vi "PosBolaFora.vi"(5 "AI Parameters":T1={"GotoKick"={"Dist do cone a frente"=150.0, "attacker farback"=1500.0, "Perto"=300.0, "min dist to kick"=150.0, "kick eps"=0.0, "Time to transition"=0.05}, "Attacker"={"CC chute"=0.09, "CC passe"=0.045, "Kick Force"=100.0, "ball-robot Kick"=200.0, "ball-robot Pass"=0.3, "drible\nAttk"=FALSE}, "Defender"={"D max"=1700.0, "Vel p/ robô av"=1000.0, "Kick Force"=100.0, "D atk-def"=0.0, "D farback"=0.0, "drible\ndef"=FALSE, "drible\ngoalie"=FALSE}, "Timeout"={"Field/v in x"=6.0, "Dist Robots"=300, "Dist up in y"=300}, "Pose Striker"={"dist"=200.0, "Numeric"=-4.0, "dist 2"=200.0, "drible\nstriker"=FALSE}, "Dist Stop"=300.0, "D ball out"=200, "D central gap "=150.0, "T pass"=0.0, "Force ++"=0.0, "range kick"=0.0, "Chute alto"=TRUE, "Marcador novo"=TRUE, "drible"=FALSE, "D drible"=300.0} {"D drible" format="%#_13g"; "D central gap" format="%#_13g"; "Dist Stop" format="%#_13g"; "Pose Striker"."Numeric" format="%#_13g"; "Defender"."Kick Force" format="%#_13g"; "Defender"."Vel p/ robô av" format="%#_13g"; "Attacker"."ball-robot Kick" format="%#_13g"; "Attacker"."Kick Force" format="%#_13g"; "Attacker"."CC passe" format="%#_13g"; "Attacker"."CC chute" format="%#_13g"; "GotoKick"."min dist to kick" format="%#_13g"; "GotoKick"."Perto" format="%#_13g"; "GotoKick"."attacker farback" format="%#_13g"; "GotoKick"."Dist do cone a frente" format="%#_13g"}, 9 "Field Size in":T2, 10 "Position da bola":dbl[](array[numeric]), 11 "Position do robot":dbl[](array[numeric])) -> (3 "Target":dbl[](array[numeric]))   [LabVIEW 2017]
uses:
  Core/Field Size.ctl
  AI Parameters.ctl
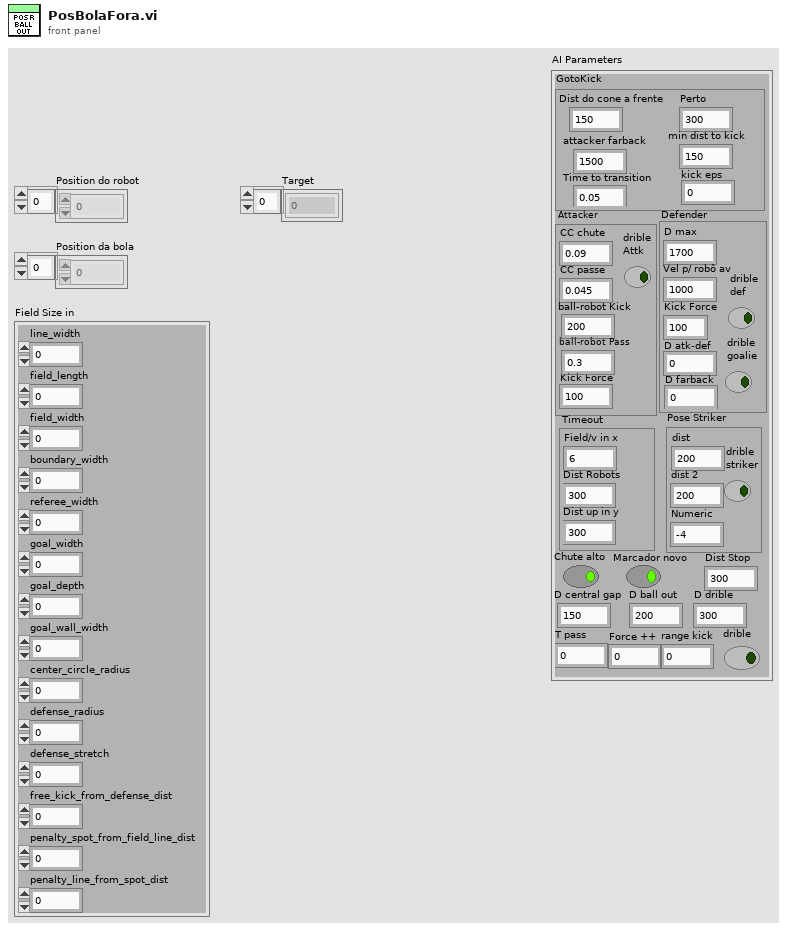
[diagram p1: front panel]
types:
  T1 = typedef "AI Parameters.ctl" = cluster{"GotoKick":cluster{"Dist do cone a frente":dbl, "attacker farback":dbl, "Perto":dbl, "min dist to kick":dbl, "kick eps":dbl, "Time to transition":dbl}, "Attacker":cluster{"CC chute":dbl, "CC passe":dbl, "Kick Force":dbl, "ball-robot Kick":dbl, "ball-robot Pass":dbl, "drible\nAttk":bool}, "Defender":cluster{"D max":dbl, "Vel p/ robô av":dbl, "Kick Force":dbl, "D atk-def":dbl, "D farback":dbl, "drible\ndef":bool, "drible\ngoalie":bool}, "Timeout":cluster{"Field/v in x":dbl, "Dist Robots":u32, "Dist up in y":u32}, "Pose Striker":cluster{"dist":dbl, "Numeric":dbl, "dist 2":dbl, "drible\nstriker":bool}, "Dist Stop":dbl, "D ball out":i32, "D central gap ":dbl, "T pass":dbl, "Force ++":dbl, "range kick":dbl, "Chute alto":bool, "Marcador novo":bool, "drible":bool, "D drible":dbl}
  T2 = typedef "Field Size.ctl" = cluster{"line_width":u32, "field_length":u32, "field_width":u32, "boundary_width":u32, "referee_width":u32, "goal_width":u32, "goal_depth":u32, "goal_wall_width":u32, "center_circle_radius":u32, "defense_radius":u32, "defense_stretch":u32, "free_kick_from_defense_dist":u32, "penalty_spot_from_field_line_dist":u32, "penalty_line_from_spot_dist":u32}
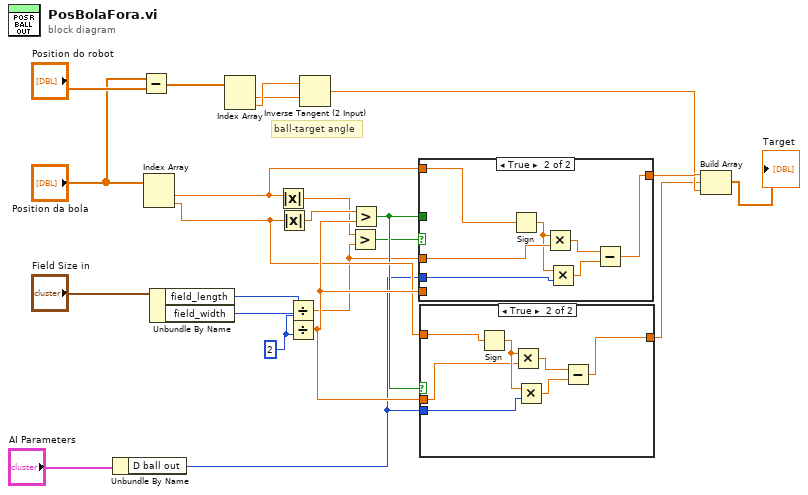
[diagram p0: block diagram]
diagram:
  w6 = u32 2 ("y")
  # "ball-target angle"
  n1 = Unbundle By Name("AI Parameters") -> ("D ball out"=w1:i32)
  n2 = Subtract(x="Position da bola", y="Position do robot") -> (x-y=w13:dbl[])
  n3 = Index Array(array="Position da bola") -> (element #1=w10:dbl, element #2=w20:dbl)  [unwired: 2 in]
  n4 = Unbundle By Name("Field Size in") -> ("field_length"=w4:u32, "field_width"=w5:u32)
  n5 = Index Array(array=w13) -> (element #1=w11:dbl, element #2=w12:dbl)  [unwired: 2 in]
  n6 = Absolute Value(x=w10) -> (abs(x)=w7:dbl)
  n7 = Absolute Value(x=w20) -> (abs(x)=w9:dbl)
  n8 = Divide(x=w4, y=w6) -> (x/y=w16:dbl)
  n9 = Divide(x=w5, y=w6) -> (x/y=w21:dbl)
  n10 = Inverse Tangent (2 Input)(1:w11, 2:w12) -> (0:w14:dbl)
  n11 = Greater?(x=w7, y=w16) -> (0:w8:bool)
  n12 = Greater?(x=w9, y=w21) -> (0:w19:bool)
  n13 = case shown="True" w8 {
    tunnel: w19 -> [_ _]
    tunnel: w10 -> [w24 w31]
    tunnel: [w24 w29] -> w15
    tunnel: w16 -> [_ w30]
    tunnel: w21 -> [_ _]
    tunnel: w1 -> [_ w25]
    frame False {
    }
    frame True {
      n14 = Sign(1:w31) -> (0:w27:dbl)
      n15 = Multiply(x=w27, y=w30) -> (x*y=w28:dbl)
      n16 = Multiply(x=w27, y=w25) -> (x*y=w26:dbl)
      n17 = Subtract(x=w28, y=w26) -> (x-y=w29:dbl)
    }
  }
  n18 = case shown="True" w19 {
    tunnel: w20 -> [w32 w36]
    tunnel: w21 -> [_ w34]
    tunnel: [w32 w35] -> w3
    tunnel: w1 -> [_ w33]
    frame False {
    }
    frame True {
      n19 = Sign(1:w36) -> (0:w38:dbl)
      n20 = Multiply(x=w38, y=w34) -> (x*y=w39:dbl)
      n21 = Multiply(x=w38, y=w33) -> (x*y=w37:dbl)
      n22 = Subtract(x=w39, y=w37) -> (x-y=w35:dbl)
    }
  }
  n23 = Build Array(w15, w3, w14) -> (→"Target":dbl[])
